vi "Avocent_match_set_command.vi"(8 "error in":errorcluster, 11 "set command":string="setport J") -> (0 "error out":errorcluster, 3 "Set switches":bool[](array[boolean])=[FALSE, FALSE, FALSE, FALSE, FALSE, FALSE, FALSE, FALSE, FALSE, TRUE, FALSE, FALSE, FALSE, FALSE, FALSE, FALSE] caption="Set Switches")   [LabVIEW 2020]
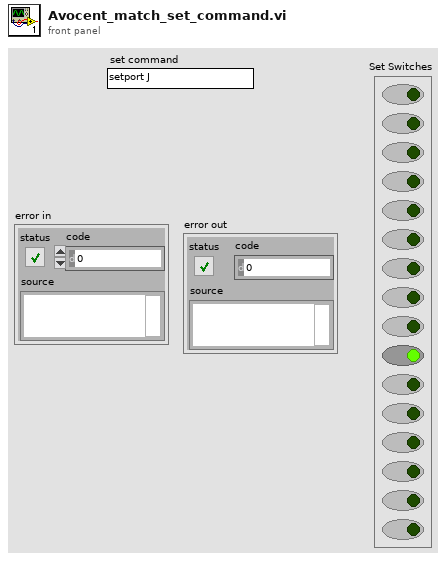
[diagram p1: front panel]
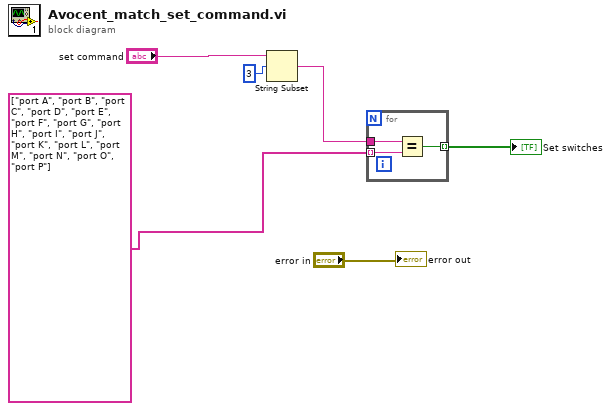
[diagram p0: block diagram]
diagram:
  n1 = String Subset(string="set command", offset (0)=3) -> (substring=w4:string)  [unwired: 1 in]
  n2 = for {
    tunnel: w4 -> [w9]
    tunnel: string[] ["port A", "port B", "port C", "port D", "port E", "port F", "port G", "port H", "port I", "port J", "port K", "port L", "port M", "port N", "port O", "port P"] ("set following Variables (empty = all avriables)") -> [w8] mode=indexing
    tunnel: [w7] -> w2 mode=indexing
    n3 = Equal?(x=w9, y=w8) -> (x = y?=w7:bool)
  }
  "Set switches" <- w2
  "error out" <- "error in"
